vi "Main.vi"(8 "error in (no error)":errorcluster, 11 "ModuleQ":refnum<queue>) -> (0 "error out":errorcluster)   [LabVIEW 2020, in "Template.lvlib"]
doc: "Use this template to build a producer/consumer design pattern with events to produce queue items. Use this design pattern instead of the User Interface Event Handler pattern for user interfaces when you want to execute code asynchronously in response to an event without slowing the user interface responsiveness."
uses:
  Template.lvlib
  Controls/QMessage.ctl
  Controls/ConsummerLoopData.ctl
  Controls/EventLoopData.ctl
panel:
  out "ModuleQ Out":refnum<queue>
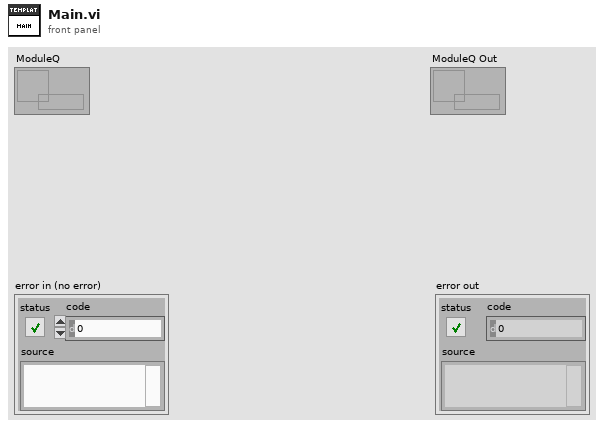
[diagram p1: front panel]
types:
  T1 = typedef "Template.lvlib/EventLoopData.ctl" = cluster{"DummyData":dbl}
  T2 = typedef "Template.lvlib/ConsummerLoopData.ctl" = cluster{"Error File Refnum":refnum<file>}
  T3 = typedef "Template.lvlib/QMessage.ctl" = cluster{"Message":string, "Data":errorcluster}
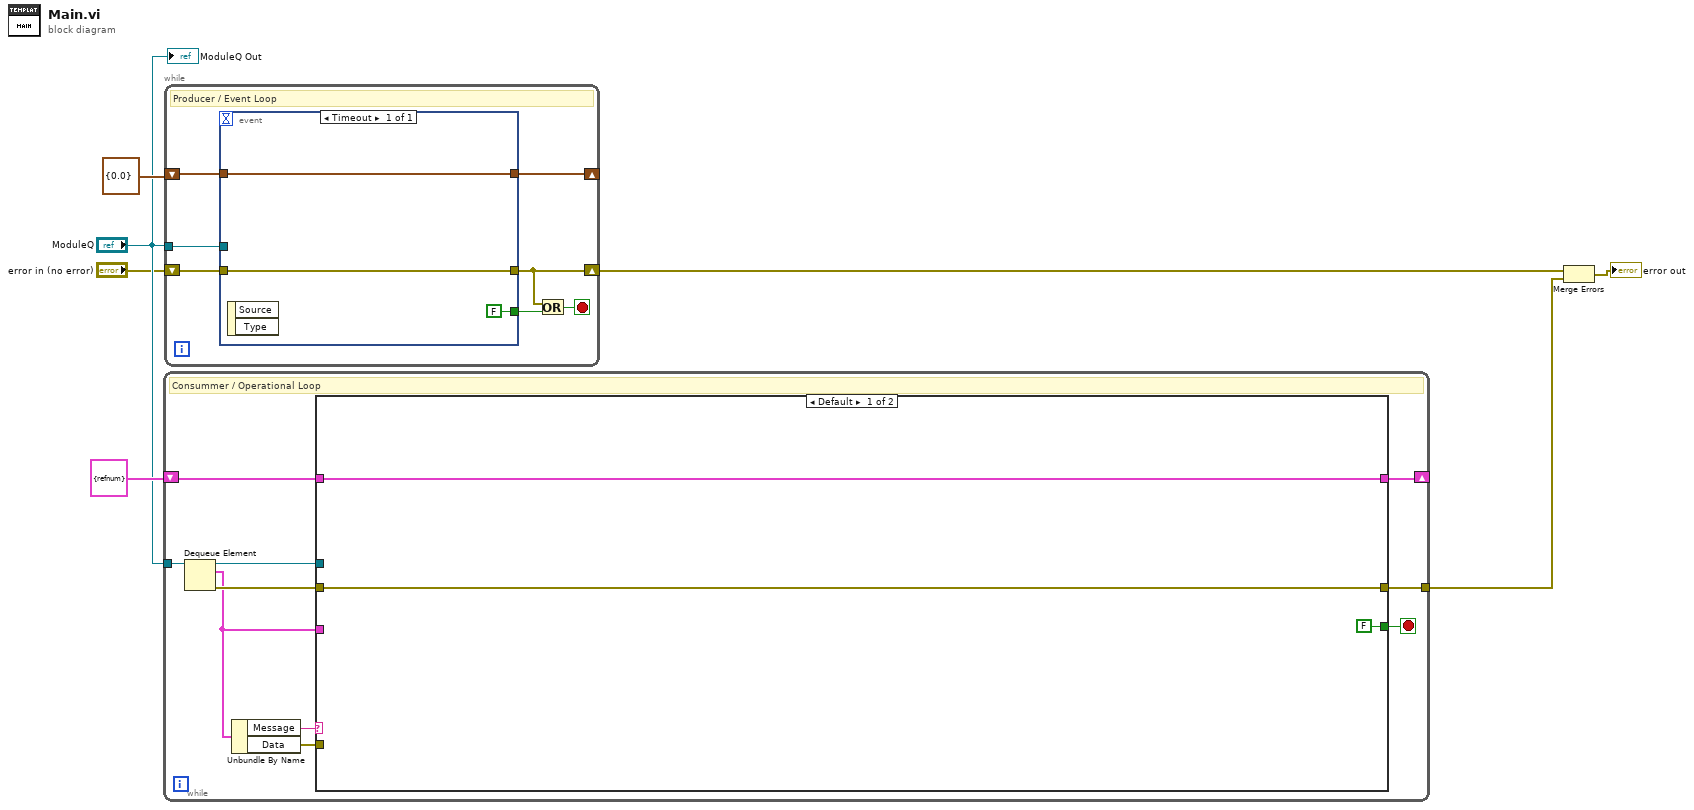
[diagram p0: block diagram]
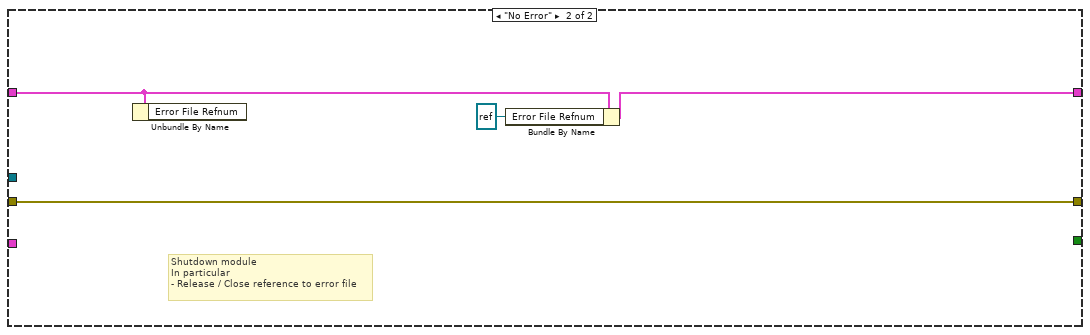
[diagram p2: hidden frame]
diagram:
  n1 = while {
    tunnel: "ModuleQ" -> [w17]
    shift-right: [w15] -> _
    shift-left: T2 {"Error File Refnum"=refnum} -> [w14]
    tunnel: [w12] -> w6
    stop <- w16 stop-if-true
    # "Consummer / Operational Loop"
    n2 = Dequeue Element(queue=w17) -> (queue out=w11:refnum<queue>, element=w10:T3, error out=w13:errorcluster)  [unwired: 2 in, 1 out]
    n3 = Unbundle By Name(w10) -> ("Message"=w9:string, "Data"=w8:errorcluster)
    n4 = case shown="Default" w9 {
      tunnel: [FALSE _] -> w16
      tunnel: [w19 w22] -> w15
      tunnel: w14 -> [w19 w23]
      tunnel: w13 -> [w18 w24]
      tunnel: [w18 w24] -> w12
      tunnel: w11 -> [_ _]
      tunnel: w10 -> [_ _]
      tunnel: w8 -> [_ _]
      frame Default {
      }
      frame "No Error" {
        # "Shutdown module\nIn particular\n- Release / Close reference to error file"
        n5 = Unbundle By Name(w23) -> ()  [unwired: 1 out]
        n6 = Bundle By Name(cluster=w23, "Error File Refnum"=refnum<file> refnum) -> (w22:T2)
      }
    }
  }
  n7 = while {
    shift-right: [w27] -> w5
    shift-left: "error in (no error)" -> [w30]
    tunnel: "ModuleQ" -> [w31]
    shift-right: [w26] -> _
    shift-left: T1 {"DummyData"=0.0} -> [w25]
    stop <- w28 stop-if-true
    # "Producer / Event Loop"
    n8 = event shown="[0] Timeout" {
      selector: _ -> [_]
      dyn-events: _ -> [_]
      timeout: _ -> [_]
      tunnel: w31 -> [_]
      tunnel: w30 -> [w33]
      tunnel: [w33] -> w27
      tunnel: [FALSE ("stop")] -> w29
      tunnel: [w34] -> w26
      tunnel: w25 -> [w34]
      event Timeout {
        n9 = event-data() -> ()  [unwired: 1 in, 2 out]
      }
    }
    n10 = Or(x=w27, y=w29) -> (x .or. y?=w28:bool)
  }
  n11 = Merge Errors(w5, w6) -> (→"error out":errorcluster)
  "ModuleQ Out" <- "ModuleQ"
